vi "Finalize.vi"(8 "error in (no error)":errorcluster, 11 "NI-XNET CAN Writer Execution Unit in":refnum<class "NI-XNET CAN Writer Execution Unit.lvclass">) -> (0 "error out":errorcluster, 3 "NI-XNET CAN Writer Execution Unit out":refnum<class "NI-XNET CAN Writer Execution Unit.lvclass">)   [LabVIEW 2020, in "Communication Bus Template Engine.lvlib" / "Implementation.lvlib" / "NI-XNET CAN Writer Execution Unit.lvclass"]
uses:
  NI-XNET CAN Writer Execution Unit.lvclass
  NI-XNET CAN Writer Execution Unit.lvclass/NI-XNET CAN Writer Execution Unit.ctl
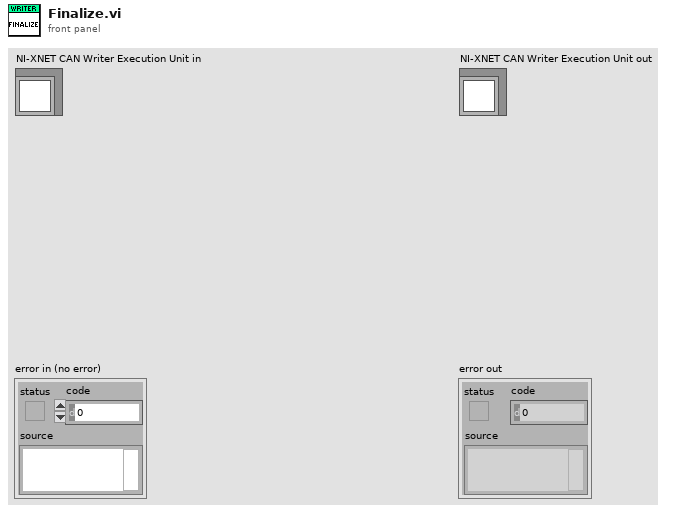
[diagram p1: front panel]
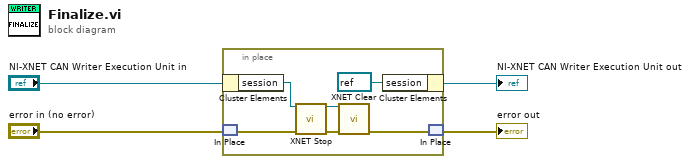
[diagram p0: block diagram]
diagram:
  n1 = in-place {
    n2 = in-place-cluster #1("NI-XNET CAN Writer Execution Unit in") -> ("session"=w8:refnum<k21>)
    n3 = in-place-match #2("error in (no error)") -> (w6:errorcluster)
    n4 = call <vilib>:"XNET Stop.vi"("session in"=w8, "error in (no error)"=w6) -> ("session out"=w10:refnum<k21>, "error out"=w9:errorcluster)  [unwired: 12 in]
    n5 = call <vilib>:"XNET Clear.vi"("session in"=w10, "error in (no error)"=w9) -> ("error out"=w5:errorcluster)  [unwired: 13 in]
    n6 = in-place-cluster #1("session"=refnum<k21> refnum) -> (→"NI-XNET CAN Writer Execution Unit out":refnum<class "NI-XNET CAN Writer Execution Unit.lvclass">)
    n7 = in-place-match #2(w5) -> (→"error out":errorcluster)
  }
